vi "Teardown.vi"(10 "Teardown":bool, 11 "Dev Actor Panel in":refnum<class "Dev Panel.lvclass">) -> (0 "error out":errorcluster)   [LabVIEW 2021, in "Dev Panel.lvclass"]
uses:
  Dev Panel.lvclass
  Dev Panel.lvclass/Dev Panel.ctl
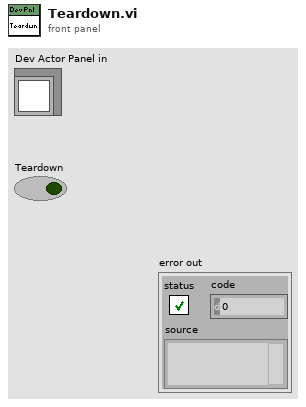
[diagram p1: front panel]
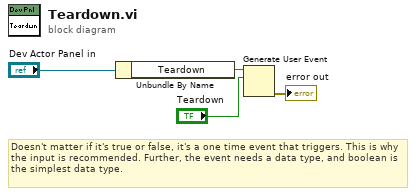
[diagram p0: block diagram]
diagram:
  # "Doesn't matter if it's true or false, it's a one time event that triggers. This is why the input is recommended. Further, the event needs a data type, and boolean is the simplest data type."
  n1 = Unbundle By Name("Dev Actor Panel in") -> ("Teardown"=w3:refnum<user-event>)
  n2 = Generate User Event(user event=w3, event data cluster="Teardown") -> (error out=→"error out":errorcluster)  [unwired: 2 in, 1 out]
